vi "Increase Accumulator.vi"(7 "reset":bool, 11 "increment":u32) -> (3 "accumulator":u32)   [LabVIEW 2017, in "Analog IO.lvlib" / "Analog Output.lvclass"]
uses:
  Analog Output.lvclass
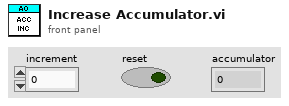
[diagram p1: front panel]
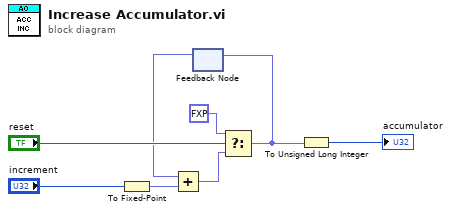
[diagram p0: block diagram]
diagram:
  n1 = To Fixed-Point(number="increment") -> (fixed-point=w5:fxp<+,32,32>)  [unwired: 1 in]
  n2 = feedback #1() -> (w1:fxp<+,32,32>)  [unwired: 1 in]
  n3 = Add(x=w1, y=w5) -> (x+y=w4:fxp<+,32,32>)
  n4 = Select(t=fxp<+,32,32> 0.0, s="reset", f=w4) -> (s? t:f=w2:fxp<+,32,32>)
  n5 = feedback-in #1(w2) -> ()
  n6 = To Unsigned Long Integer(number=w2) -> (unsigned 32bit integer=→"accumulator":u32)
